vi "4Pi 4Pi Modes - Mode Scan Data AE.vi"(0 "Amplitude":dbl[](array[numeric]), 2 "Action":T1, 11 "Metric":dbl[](array[numeric])) -> (4 "Amplitude Out":dbl[](array[numeric]), 15 "Metric Out":dbl[](array[numeric]))   [LabVIEW 2016]
uses:
  4Pi 4Pi Modes - Controls/4Pi 4Pi Modes - Standard Action.ctl
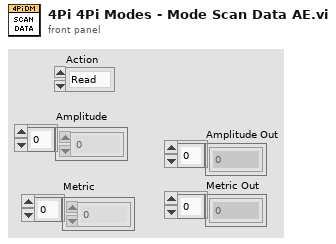
[diagram p1: front panel]
types:
  T1 = typedef "4Pi 4Pi Modes - Standard Action.ctl" = enum16{"Read", "Write"}
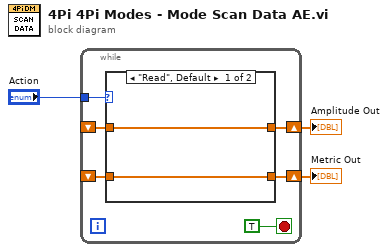
[diagram p0: block diagram]
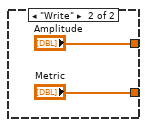
[diagram p2: hidden frame]
diagram:
  n1 = while {
    tunnel: "Action" -> [w8]
    shift-right: [w7] -> w2
    shift-left: _ -> [w5]
    shift-right: [w6] -> w1
    shift-left: _ -> [w4]
    stop <- TRUE stop-if-true
    n2 = case shown="\"Read\", Default" w8 {
      tunnel: [w11 "Amplitude"] -> w7
      tunnel: [w10 "Metric"] -> w6
      tunnel: w5 -> [w11 _]
      tunnel: w4 -> [w10 _]
      frame "Read", Default {
      }
      frame "Write" {
      }
    }
  }
  "Amplitude Out" <- w2
  "Metric Out" <- w1
